vi "SerialBusHound.vi"() -> ()   [LabVIEW 2011]
uses:
  Enumerator/CmdType.ctl
  <vilib>/Platform/TimedLoop/XDataNode/timing_clust.ctl
  <vilib>/Platform/TimedLoop/XDataNode/nitl_modes.ctl
  <vilib>/Platform/TimedLoop/XDataNode/wakeup.ctl
  Variable/gSTOP.vi
  <vilib>/Platform/TimedLoop/XDataNode/XDataNode.xnode
  <vilib>/Platform/TimedLoop/XDataNode/XDNodeRunTimeDep.lvlib
panel:
  in  "Out Packet":bool=TRUE
  in  "In Packet":bool=TRUE
  in  "Dispaly":bool=TRUE
  in  "Cmd Type":T1=enum."EventPolling"
  out "Time Stamp":timestamp format="%<%H:%M:%S\n%d/%m/%Y>T"
  in  "com port":refnum<visa-resource-name>="COM4"
  in  "parity":u16(ring) items=["None", "Odd", "Even", "Mark", "Space"]
  in  "data bits":u16(ring)=8 items=["5"=5, "6"=6, "7"=7, "8"=8]
  in  "stop bits":u16(ring)=10 items=["1.0"=10, "1.5"=15, "2.0"=20]
  out "Card Info":string="25469:57693"
  out "status":bool
  in  "baud rate":u32=9600
  in  "run":bool
  out "Slide":i32(slide)=67 scale=0.0..100.0
  in  "Multicolumn Listbox":i32(listbox)=66
  # "Serial Settings"
  # "Card Information"
  # "Com Port :"
  # "Status :"
  # "Parity :"
  # "Stop Bits :"
  # "Baud Rate :"
  # "Data Bits :"
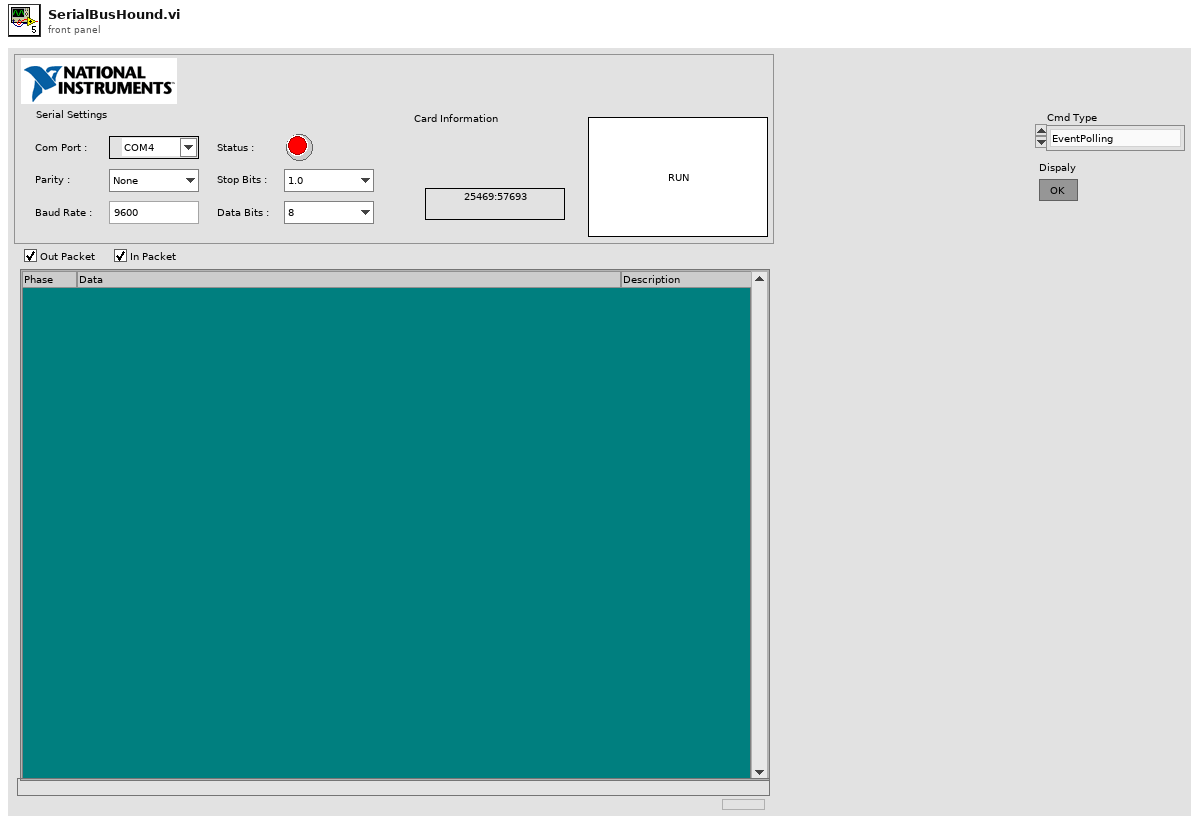
[diagram p1: front panel]
types:
  T1 = typedef "CmdType.ctl" = enum16{"GetEventLog", "DelTransaction", "InvalidMessage", "RelayControl", "RelayOff", "RelayOn", "VaildMessage", "EventPolling", "StoppingWaiting", "PromptKeying-in"}
  T2 = enum16{"Obtain", "Enqueue", "Dequeue", "Release"}
  T3 = enum16{"Open", "R", "W", "R->W", "W->R", "Close"}
  T4 = typedef "XDNodeRunTimeDep.lvlib/timing_clust.ctl" = cluster{"Expected End [f-1]":u64, "Actual End [f-1]":u64, "Finished Late? [f-1]":bool, "Expected End [i-1]":u64, "Actual End [i-1]":u64, "Finished Late? [i-1]":bool, "Expected Start [i]":u64, "Actual Start [i]":u64, "Expected Start [f]":u64, "Actual Start [f]":u64, "Source Name":string, "Structure Name":string, "Period":i64, "Deadline":i64, "Offset":i64, "Start":i64, "Priority":i32, "Timeout":i32, "Mode":T5, "Wakeup Reason":T6, "Error":errorcluster, "Source Type":string, "Secondary Source Type":string, "Global End Time":u64, "Global Start Time":u64, "Frame Duration":u64, "Iteration Duration":u64, "Assigned CPU":i32, "I/O Scan Engine Mode":u32}
  T5 = typedef "XDNodeRunTimeDep.lvlib/nitl_modes.ctl" = enum32{"No Change", "Process missed periods, maintain original phase", "Discard missed periods, maintain original phase", "Process missed periods, ignore original phase", "Discard missed periods, ignore original phase"}
  T6 = typedef "XDNodeRunTimeDep.lvlib/wakeup.ctl" = enum32{"Normal", "Aborted", "Asynchronous wakeup", "Timing source error", "Timed loop error", "Timeout"}
  T7 = cluster{"VISA-RS232":refnum<visa-resource-name>, "baud rate":u32, "data bits":u16, "parity":u16, "stop bits":u16}
  T8 = typedef "LVRectTypeDef.ctl" = cluster{"left":i16, "top":i16, "right":i16, "bottom":i16}
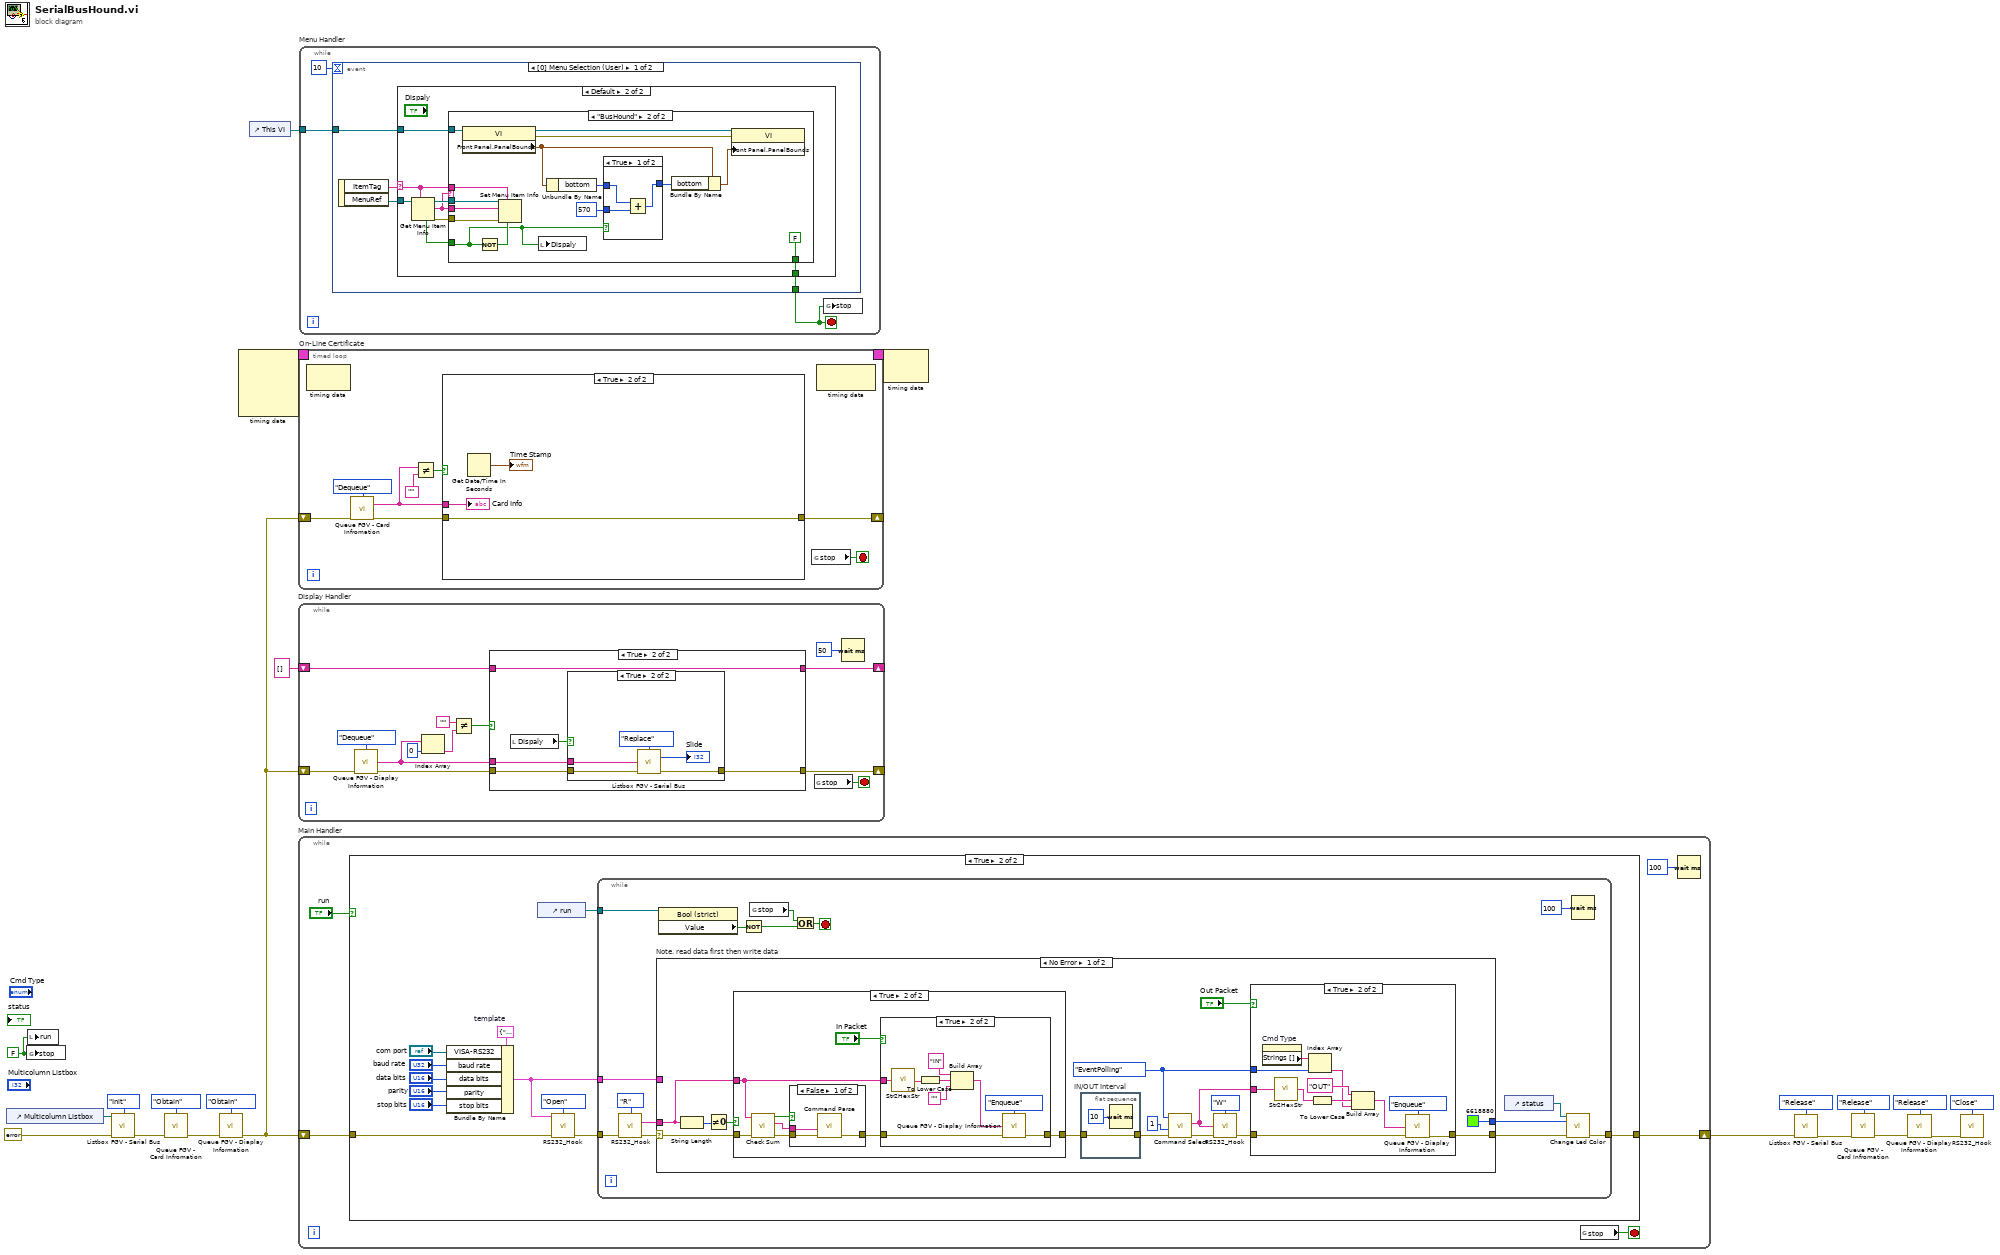
[diagram p0: block diagram]
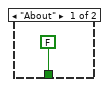
[diagram p5: hidden frame]
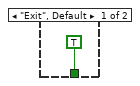
[diagram p6: hidden frame]
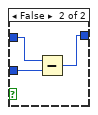
[diagram p7: hidden frame]
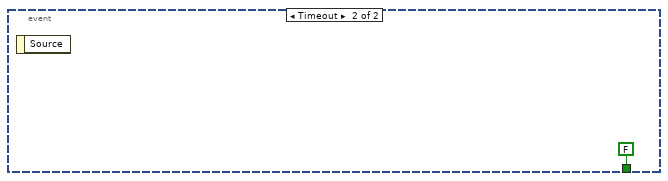
[diagram p8: hidden frame]
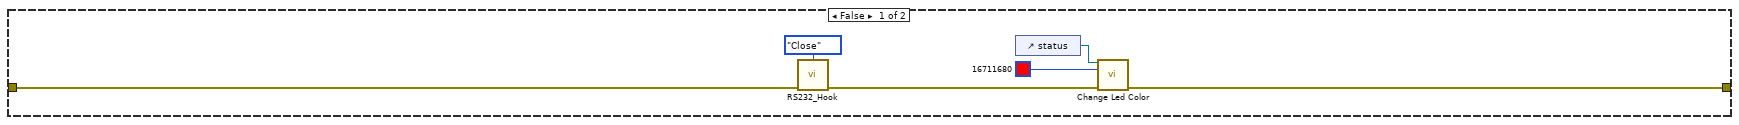
[diagram p9: hidden frame]
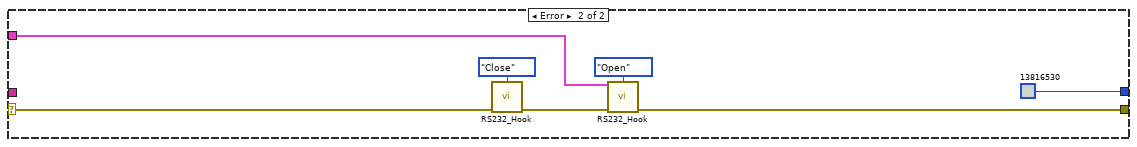
[diagram p14: hidden frame]
diagram:
  w6 = FALSE ("stop")
  n1 = control-ref of="Multicolumn Listbox"() -> (w16:refnum<vi>)
  n2 = global write "gSTOP.vi" "stop"(w6) -> ()
  n3 = local write "run"(w6) -> ()
  n4 = call "Listbox FGV - Serial Bus.vi"("MulticolumnListbox in"=w16, "Enum"=enum16{"Init", "Replace", "Clear", "Release"}."Init", "error in"=errorcluster {"status"=FALSE, "code"=0, "source"=""} ("error constant")) -> ("error out"=w8:errorcluster)  [unwired: 11 in, 1 out]
  n5 = call "Queue FGV - Card Infromation.vi"("Mode"=T2."Obtain", "error in (no error)"=w8) -> ("error out"=w14:errorcluster)  [unwired: 12 in, 1 out]
  n6 = call "Queue FGV - Diaplay Information.vi"("Mode"=T2."Obtain", "error in (no error)"=w14) -> ("error out"=w13:errorcluster)  [unwired: 12 in, 1 out]
  n7 = node-c288() -> (w19:T4)  [unwired: 4 in]
  n8 = control-ref of="This VI"() -> (w7:refnum<vi>)
  n9 = while "Display Handler" {
    shift-right: [w31] -> _
    shift-left: w13 -> [w33]
    shift-right: [w22] -> _
    shift-left: string[] [] ("Queue Out") -> [w23]
    stop <- w30 stop-if-true
    n10 = call "Queue FGV - Diaplay Information.vi"("Mode"=T2."Dequeue", "error in (no error)"=w33) -> ("Queue Out"=w24:string[], "error out"=w32:errorcluster)  [unwired: 12 in]
    n11 = Index Array(array=w24, index=0) -> (element=w27:string)
    n12 = Not Equal?(x="", y=w27) -> (x != y?=w25:bool)
    n13 = case shown="True" w25 {
      tunnel: w32 -> [w36 w41]
      tunnel: [w36 w40] -> w31
      tunnel: w24 -> [_ w39]
      tunnel: w23 -> [w35 w38]
      tunnel: [w35 w38] -> w22
      frame False {
      }
      frame True {
        n14 = local read "Dispaly"() -> (w37:bool)
        n15 = case shown="True" w37 {
          tunnel: w41 -> [w42 w47]
          tunnel: [w42 w46] -> w40
          tunnel: w39 -> [_ w45]
          frame False {
          }
          frame True {
            n16 = call "Listbox FGV - Serial Bus.vi"("Enum"=enum16{"Init", "Replace", "Clear", "Release"}."Replace", "Array"=w45, "error in"=w47) -> ("Index"=→"Slide":i32, "error out"=w46:errorcluster)  [unwired: 11 in]
          }
        }
      }
    }
    n17 = global read "gSTOP.vi" "stop"() -> (w30:bool)
    n18 = Wait (ms)(milliseconds to wait=u32 50 ("ms")) -> ()  [unwired: 1 out]
  }
  n19 = while "Main Handler" {
    shift-right: [w49] -> w2
    shift-left: w13 -> [w52]
    stop <- w51 stop-if-true
    n20 = case shown="True" "run" {
      tunnel: w52 -> [w57 w64]
      tunnel: [w54 w70] -> w49
      frame False {
        n21 = call "RS232_Hook.vi"("Mode"=T3."Close", "error in"=w57) -> ("error out"=w55:errorcluster)  [unwired: 12 in, 1 out]
        n22 = control-ref of="status"() -> (w56:refnum<vi>)
        n23 = call "Change Led Color.vi"("Boolean in"=w56, "Color Box"=u32 16711680, "error in (no error)"=w55) -> ("error out"=w54:errorcluster)  [unwired: 12 in]
      }
      frame True {
        w68 = T7 {"VISA-RS232"="", "baud rate"=0, "data bits"=0, "parity"=0, "stop bits"=0}  # template
        n24 = Bundle By Name(cluster=w68, "VISA-RS232"="com port", "baud rate"="baud rate", "data bits"="data bits", "parity"="parity", "stop bits"="stop bits") -> (w65:T7)
        n25 = control-ref of="run"() -> (w63:refnum<vi>)
        n26 = call "RS232_Hook.vi"("RS232 Config"=w65, "Mode"=T3."Open", "error in"=w64) -> ("error out"=w66:errorcluster)  [unwired: 11 in, 1 out]
        n27 = while {
          tunnel: [w72] -> w70
          tunnel: w66 -> [w85]
          tunnel: w65 -> [w84]
          tunnel: w63 -> [w80]
          stop <- w78 stop-if-true
          n28 = call "RS232_Hook.vi"("Mode"=T3."R", "error in"=w85) -> ("data out"=w82:string, "error out"=w83:errorcluster)  [unwired: 12 in]
          n29 = case "Note. read data first then write data" shown="No Error" w83 {
            selector: w83 -> [w93 w142]
            tunnel: [w91 w140] -> w73
            tunnel: w84 -> [_ w139]
            tunnel: w82 -> [w100 _]
            tunnel: [u32 6618880 u32 13816530] -> w74
            frame No Error {
              w89 = CmdType."EventPolling" ("Cmd Type")
              n30 = String Length(string=w100) -> (length=w95:i32)
              n31 = Not Equal To 0?(x=w95) -> (x != 0?=w94:bool)
              n32 = case shown="True" w94 {
                tunnel: w100 -> [_ w117]
                tunnel: w93 -> [w115 w120]
                tunnel: [w115 w118] -> w88
                frame False {
                }
                frame True {
                  n33 = call "Check Sum.vi"("error in (no error)"=w120, "string in"=w117) -> ("error out"=w121:errorcluster, "string out"=w123:string, "No Parse"=w122:bool)  [unwired: 7 in]
                  n34 = case shown="False" w122 {
                    tunnel: w121 -> [w136 w137]
                    tunnel: [w135 w137] -> w119
                    tunnel: w123 -> [w134 _]
                    frame False {
                      n35 = call "Command Parse.vi"("error in (no error)"=w136, "Read Buffer"=w134) -> ("error out"=w135:errorcluster)  [unwired: 9 in]
                    }
                    frame True {
                    }
                  }
                  n36 = case shown="True" "In Packet" {
                    tunnel: w119 -> [w124 w132]
                    tunnel: [w124 w131] -> w118
                    tunnel: w117 -> [_ w126]
                    frame False {
                    }
                    frame True {
                      n37 = call "Str2HexStr.vi"("data out"=w126) -> ("String"=w128:string)  [unwired: 14 in]
                      n38 = To Lower Case(string=w128) -> (all lower case string=w127:string)
                      n39 = Build Array("IN", w127, "") -> (w129:string[])
                      n40 = call "Queue FGV - Diaplay Information.vi"("Mode"=T2."Enqueue", "Queue In"=w129, "error in (no error)"=w132) -> ("error out"=w131:errorcluster)  [unwired: 11 in, 1 out]
                    }
                  }
                }
              }
              n41 = flat-sequence "IN/OUT Interval" {
                tunnel: w88 -> [w101]
                tunnel: [w101] -> w87
                frame #0 {
                  n42 = Wait (ms)(milliseconds to wait=u32 10 ("ms")) -> ()  [unwired: 1 out]
                }
              }
              n43 = call "Command Select.vi"("error in (no error)"=w87, "Node Id"=u8 1, "Cmd Type"=w89) -> ("error out"=w98:errorcluster, "Cmd Str"=w90:string)  [unwired: 7 in]
              n44 = call "RS232_Hook.vi"("Mode"=T3."W", "data in"=w90, "error in"=w98) -> ("error out"=w92:errorcluster)  [unwired: 11 in, 1 out]
              n45 = case shown="True" "Out Packet" {
                tunnel: w92 -> [w103 w114]
                tunnel: [w103 w113] -> w91
                tunnel: w90 -> [_ w107]
                tunnel: w89 -> [_ w104]
                frame False {
                }
                frame True {
                  n46 = property on="Cmd Type" class="Enum (strict)"() -> ("Strings []"=w106:string[])  [unwired: 2 in, 2 out]
                  n47 = call "Str2HexStr.vi"("data out"=w107) -> ("String"=w108:string)  [unwired: 14 in]
                  n48 = Index Array(array=w106, index=w104) -> (element=w105:string)
                  n49 = To Lower Case(string=w108) -> (all lower case string=w109:string)
                  n50 = Build Array("OUT", w109, w105) -> (w110:string[])
                  n51 = call "Queue FGV - Diaplay Information.vi"("Mode"=T2."Enqueue", "Queue In"=w110, "error in (no error)"=w114) -> ("error out"=w113:errorcluster)  [unwired: 11 in, 1 out]
                }
              }
            }
            frame Error {
              n52 = call "RS232_Hook.vi"("Mode"=T3."Close", "error in"=w142) -> ("error out"=w141:errorcluster)  [unwired: 12 in, 1 out]
              n53 = call "RS232_Hook.vi"("RS232 Config"=w139, "Mode"=T3."Open", "error in"=w141) -> ("error out"=w140:errorcluster)  [unwired: 11 in, 1 out]
            }
          }
          n54 = property class="Bool (strict)"(reference=w80) -> ("Value"=w79:bool)  [unwired: 1 in, 2 out]
          n55 = Not(x=w79) -> (.not. x?=w76:bool)
          n56 = global read "gSTOP.vi" "stop"() -> (w77:bool)
          n57 = Or(x=w77, y=w76) -> (x .or. y?=w78:bool)
          n58 = control-ref of="status"() -> (w75:refnum<vi>)
          n59 = call "Change Led Color.vi"("Boolean in"=w75, "Color Box"=w74, "error in (no error)"=w73) -> ("error out"=w72:errorcluster)  [unwired: 12 in]
          n60 = Wait (ms)(milliseconds to wait=u32 100 ("ms")) -> ()  [unwired: 1 out]
        }
      }
    }
    n61 = global read "gSTOP.vi" "stop"() -> (w51:bool)
    n62 = Wait (ms)(milliseconds to wait=u32 100 ("ms")) -> ()  [unwired: 1 out]
  }
  n63 = timed-loop "On-Line Certificate" {
    shift-right: [w148] -> _
    shift-left: w13 -> [w151]
    timing: w19 -> [_]
    timing-out: [_] -> w18
    stop <- w146 stop-if-true
    n64 = node-c288() -> ()  [unwired: 1 in, 1 out]
    n65 = call "Queue FGV - Card Infromation.vi"("Mode"=T2."Dequeue", "error in (no error)"=w151) -> ("Queue Out"=w145:string, "error out"=w149:errorcluster)  [unwired: 12 in]
    n66 = Not Equal?(x=w145, y="") -> (x != y?=w150:bool)
    n67 = case shown="True" w150 {
      tunnel: w149 -> [w155 w158]
      tunnel: [w155 w158] -> w148
      tunnel: w145 -> [_ w157]
      frame False {
      }
      frame True {
        n68 = Get Date/Time In Seconds() -> (seconds since 1Jan1904=→"Time Stamp":timestamp)
        "Card Info" <- w157
      }
    }
    n69 = global read "gSTOP.vi" "stop"() -> (w146:bool)
    n70 = node-c288() -> ()  [unwired: 1 in, 1 out]
  }
  n71 = while "Menu Handler" {
    tunnel: w7 -> [w159]
    stop <- w161 stop-if-true
    n72 = event shown="[0] Menu Selection (User)" {
      selector: _ -> [_ _]
      dyn-events: _ -> [_ _]
      timeout: 10 -> [_ _]
      tunnel: [w163 FALSE] -> w161
      tunnel: w159 -> [w162 _]
      event Menu Selection (User) {
        n73 = event-data() -> ("ItemTag"=w164:string, "MenuRef"=w165:refnum<k9>)  [unwired: 1 in]
        n74 = case shown="Default" w164 {
          selector: w164 -> [_ w168]
          tunnel: w165 -> [_ w174]
          tunnel: [FALSE w173] -> w163
          tunnel: w162 -> [_ w167]
          frame "About" {
          }
          frame Default {
            n75 = Get Menu Item Info(7:w168, 11:w174) -> (0:w170:errorcluster, 2:w169:string, 3:w172:refnum<k9>, 4:w171:bool)  [unwired: 1 in, 3 out]
            n76 = case shown="\"BusHound\"" w169 {
              tunnel: [TRUE FALSE] -> w173
              tunnel: w172 -> [_ w187]
              tunnel: w171 -> [_ w176]
              tunnel: w170 -> [_ w189]
              tunnel: w169 -> [_ w186]
              tunnel: w168 -> [_ w185]
              tunnel: w167 -> [_ w178]
              frame "Exit", Default {
              }
              frame "BusHound" {
                n77 = property class="VI"(reference=w178) -> (reference out=w184:refnum<vi>, error out=w183:errorcluster, "Front Panel.PanelBounds"=w182:T8)  [unwired: 1 in]
                n78 = Not(x=w176) -> (.not. x?=w188:bool)
                n79 = Set Menu Item Info(6:w188, 7:w185, 8:w189, 10:w186, 11:w187) -> ()  [unwired: 2 in, 2 out]
                n80 = local write "Dispaly"(w176) -> ()
                n81 = Unbundle By Name(w182) -> ("bottom"=w180:i16)
                n82 = case shown="True" w176 {
                  tunnel: w180 -> [w193 w196]
                  tunnel: [w192 w195] -> w179
                  tunnel: i16 570 ("y") -> [w191 w194]
                  frame True {
                    n83 = Add(x=w193, y=w191) -> (x+y=w192:i16)
                  }
                  frame False {
                    n84 = Subtract(x=w196, y=w194) -> (x-y=w195:i16)
                  }
                }
                n85 = Bundle By Name(cluster=w182, "bottom"=w179) -> (w181:T8)
                n86 = property class="VI"(reference=w184, error in=w183, "Front Panel.PanelBounds"=w181) -> ()  [unwired: 2 out]
              }
            }
          }
        }
      }
      event Timeout {
        n87 = event-data() -> ()  [unwired: 1 in, 1 out]
      }
    }
    n88 = global write "gSTOP.vi" "stop"(w161) -> ()
  }
  n89 = node-c288(w18) -> ()  [unwired: 1 out]
  n90 = call "Listbox FGV - Serial Bus.vi"("Enum"=enum16{"Init", "Replace", "Clear", "Release"}."Release", "error in"=w2) -> ("error out"=w1:errorcluster)  [unwired: 12 in, 1 out]
  n91 = call "Queue FGV - Card Infromation.vi"("Mode"=T2."Release", "error in (no error)"=w1) -> ("error out"=w11:errorcluster)  [unwired: 12 in, 1 out]
  n92 = call "Queue FGV - Diaplay Information.vi"("Mode"=T2."Release", "error in (no error)"=w11) -> ("error out"=w10:errorcluster)  [unwired: 12 in, 1 out]
  n93 = call "RS232_Hook.vi"("Mode"=T3."Close", "error in"=w10) -> ()  [unwired: 12 in, 2 out]
